vi "Falling Edge Detector.vi"(1 "Signal In":bool) -> (0 "Edge Detected?":bool)   [LabVIEW 2012]
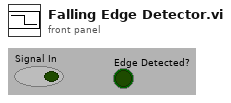
[diagram p1: front panel]
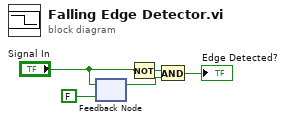
[diagram p0: block diagram]
diagram:
  n1 = feedback-in #1("Signal In") -> ()
  n2 = feedback #1(FALSE) -> (w1:bool)
  n3 = Not(x="Signal In") -> (.not. x?=w3:bool)
  n4 = And(x=w3, y=w1) -> (x .and. y?=→"Edge Detected?":bool)
